vi "LSMcontroller_v61_updatedROIselection.vi"() -> ()   [LabVIEW 2015] (continued)
                    n3057 = Build Path(base path=w6251, name or relative path="subVIs\\Image\\SetROI_v4.vi") -> (appended path=w6249:path)
                    n3058 = call <vilib>:"Set Busy.vi"() -> ("error out"=w6247:errorcluster)  [unwired: 10 in, 1 out]
                    n3059 = Open VI Reference(type specifier VI Refnum (for type only)=refnum<vi> refnum, vi path=w6249, error in (no error)=w6247) -> (vi reference=w6245:refnum<vi>, error out=w6243:errorcluster)  [unwired: 3 in]
                    n3060 = call-by-ref "?"(reference=w6245, error in=w6243) -> (reference out=w6244:refnum<vi>, error out=w6242:errorcluster)  [unwired: 1 in]
                    n3061 = Close Reference(reference=w6244, error in (no error)=w6242) -> (error out=w6246:errorcluster)
                    n3062 = call <vilib>:"Unset Busy.vi"("error in (no error)"=w6246) -> ()  [unwired: 10 in, 1 out]
                    n3063 = local write "status"(w6246) -> ()
                  }
                  frame #2 {
                    n3064 = call "2pparameters.vi"("command"="get") -> ("params out"=w6276:T11)  [unwired: 1 in]
                    n3065 = Unbundle By Name(w6276) -> ("Xpixels Img"=w6275:i32, "Vx-min Img"=w6274:dbl, "VX-max Img"=w6273:dbl, "Ypixels Img"=w6272:i32, "Vy-min Img"=w6271:dbl, "Vy-max Img"=w6270:dbl, "Colormap"=w6269:u16, "square pixels"=w6268:bool, "square matrix"=w6267:bool, "Angle Img"=w6266:dbl, "Drawing Mode"=w6265:u16)
                    n3066 = local write "xpixels ref"(w6275) -> ()
                    n3067 = local write "Vx-min ref"(w6274) -> ()
                    n3068 = local write "Vx-max ref"(w6273) -> ()
                    n3069 = local write "ypixels ref"(w6272) -> ()
                    n3070 = local write "Vy-min ref"(w6271) -> ()
                    n3071 = local write "Vy-max ref"(w6270) -> ()
                    n3072 = local write "Colormap"(w6269) -> ()
                    n3073 = local write "Square pixels"(w6268) -> ()
                    n3074 = local write "square matrix"(w6267) -> ()
                    n3075 = local write "Angle ref"(w6266) -> ()
                    n3076 = local write "ROI Type"(w6265) -> ()
                    n3077 = call "2pparameters.vi"("command"="get") -> ("params out"=w6259:T11)  [unwired: 1 in]
                    n3078 = Unbundle By Name(w6259) -> ("Xpixels"=w6253:i32, "Vxminref"=w6257:dbl, "Vxmaxref"=w6256:dbl, "Ypixels"=w6252:i32, "Vyminref"=w6255:dbl, "Vymaxref"=w6254:dbl, "Colormap"=w6260:u16, "square pixels"=w6261:bool, "square matrix"=w6262:bool, "Angle draw"=w6263:dbl, "Drawing Mode"=w6264:u16)
                    n3079 = local write "Vy-max draw"(w6254) -> ()
                    n3080 = local write "Angle drawing"(w6263) -> ()
                    n3081 = local write "Colormap"(w6260) -> ()
                    n3082 = local write "Square pixels"(w6261) -> ()
                    n3083 = local write "square matrix"(w6262) -> ()
                    n3084 = local write "ROI Type"(w6264) -> ()
                    n3085 = local write "xpixels draw"(w6253) -> ()
                    n3086 = local write "ypixels draw"(w6252) -> ()
                    n3087 = local write "Vx-min draw"(w6257) -> ()
                    n3088 = local write "Vx-max draw"(w6256) -> ()
                    n3089 = local write "Vy-min draw"(w6255) -> ()
                  }
                  frame #3 {
                    n3090 = property on="ROI" class="Bool (strict)"("Val(Sgnl)"=FALSE ("x/y scan")) -> ()  [unwired: 2 in, 2 out]
                  }
                }
              }
            }
          }
          event "Xdattype": Value Change {
            n3091 = event-data() -> ()  [unwired: 1 in, 1 out]
            n3092 = case shown="True" "Xdattype" {
              frame False {
              }
              frame True {
                n3093 = stacked-sequence {
                  frame #0 {
                    n3094 = Current VI's Path() -> (path=w6289:path)
                    n3095 = Strip Path(path=w6289) -> (stripped path=w6290:path)  [unwired: 1 out]
                    n3096 = Build Path(base path=w6290, name or relative path="subVIs\\Misc\\Changedataconfig.vi") -> (appended path=w6288:path)
                    n3097 = call <vilib>:"Set Busy.vi"() -> ("error out"=w6286:errorcluster)  [unwired: 10 in, 1 out]
                    n3098 = Open VI Reference(type specifier VI Refnum (for type only)=refnum<vi> refnum, vi path=w6288, error in (no error)=w6286) -> (vi reference=w6281:refnum<vi>, error out=w6283:errorcluster)  [unwired: 3 in]
                    n3099 = call-by-ref "?"(reference=w6281, error in=w6283) -> (reference out=w6285:refnum<vi>, error out=w6284:errorcluster)  [unwired: 12 in]
                    n3100 = Close Reference(reference=w6285, error in (no error)=w6284) -> (error out=w6280:errorcluster)
                    "status" <- w6280
                    n3101 = call <vilib>:"Unset Busy.vi"("error in (no error)"=w6280) -> ()  [unwired: 10 in, 1 out]
                  }
                  frame #1 {
                    n3102 = property on="Xdattype" class="Bool (strict)"("Val(Sgnl)"=FALSE ("x/y scan")) -> ()  [unwired: 2 in, 2 out]
                  }
                }
              }
            }
          }
          event "XautoOD": Value Change {
            n3103 = event-data() -> ()  [unwired: 1 in, 1 out]
            n3104 = case shown="True" "XautoOD" {
              frame False {
              }
              frame True {
                n3105 = stacked-sequence {
                  frame #0 {
                    n3106 = Current VI's Path() -> (path=w6302:path)
                    n3107 = Strip Path(path=w6302) -> (stripped path=w6303:path)  [unwired: 1 out]
                    n3108 = Build Path(base path=w6303, name or relative path="subVIs\\Misc\\ChangeautoODs.vi") -> (appended path=w6301:path)
                    n3109 = call <vilib>:"Set Busy.vi"() -> ("error out"=w6299:errorcluster)  [unwired: 10 in, 1 out]
                    n3110 = Open VI Reference(type specifier VI Refnum (for type only)=refnum<vi> refnum, vi path=w6301, error in (no error)=w6299) -> (vi reference=w6294:refnum<vi>, error out=w6296:errorcluster)  [unwired: 3 in]
                    n3111 = call-by-ref "?"(reference=w6294, error in=w6296) -> (reference out=w6298:refnum<vi>, error out=w6297:errorcluster)  [unwired: 12 in]
                    n3112 = Close Reference(reference=w6298, error in (no error)=w6297) -> (error out=w6293:errorcluster)
                    "status 2" <- w6293
                    n3113 = call <vilib>:"Unset Busy.vi"("error in (no error)"=w6293) -> ()  [unwired: 10 in, 1 out]
                  }
                  frame #1 {
                    n3114 = property on="XautoOD" class="Bool (strict)"("Val(Sgnl)"=FALSE ("x/y scan")) -> ()  [unwired: 2 in, 2 out]
                  }
                }
              }
            }
          }
          event "SetMan": Value Change {
            n3115 = event-data() -> ()  [unwired: 1 in, 1 out]
            n3116 = case shown="True" "SetMan" {
              frame False {
              }
              frame True {
                n3117 = stacked-sequence {
                  frame #0 {
                    w6306 = u16 0 items=["Rectangle", "Circle", "Freeform Boundary", "Freeform Interior"] ("ROI Type")
                    n3118 = local write "ROI Type"(w6306) -> ()
                    n3119 = local read "Square pixels"() -> (w6312:bool)
                    n3120 = case shown="True" w6312 {
                      frame False {
                        n3121 = local read "square matrix"() -> (w6313:bool)
                        n3122 = case shown="False" w6313 {
                          frame False {
                            "ypixels ref" <- "ypixels"
                            "xpixels ref" <- "xpixels"
                          }
                          frame True {
                            n3123 = local read "xpixels"() -> (w6318:i32)
                            n3124 = local read "ypixels"() -> (w6317:i32)
                            n3125 = Max & Min(x=w6318, y=w6317) -> (max(x,y)=w6316:i32)  [unwired: 1 out]
                            n3126 = local write "xpixels ref"(w6316) -> ()
                            n3127 = local write "ypixels ref"(w6316) -> ()
                          }
                        }
                      }
                      frame True {
                        n3128 = local read "square matrix"() -> (w6319:bool)
                        n3129 = case shown="False" w6319 {
                          frame False {
                            n3130 = local read "Vxmax"() -> (w6333:dbl)
                            n3131 = local read "Vx-min"() -> (w6332:dbl)
                            n3132 = local read "Vy-max"() -> (w6328:dbl)
                            n3133 = local read "Vy-min"() -> (w6329:dbl)
                            n3134 = Subtract(x=w6328, y=w6329) -> (x-y=w6330:dbl)
                            n3135 = Subtract(x=w6333, y=w6332) -> (x-y=w6331:dbl)
                            n3136 = Absolute Value(x=w6330) -> (abs(x)=w6321:dbl)
                            n3137 = Absolute Value(x=w6331) -> (abs(x)=w6322:dbl)
                            n3138 = Divide(x=w6322, y=w6321) -> (x/y=w6327:dbl)
                            n3139 = Greater Or Equal?(x=w6322, y=w6321) -> (x >= y?=w6320:bool)
                            n3140 = local read "xpixels"() -> (w6326:i32)
                            n3141 = local read "ypixels"() -> (w6323:i32)
                            n3142 = case shown="False" w6320 {
                              tunnel: w6327 -> [w6338 w6341]
                              tunnel: w6326 -> [w6335 _]
                              tunnel: [w6335 w6340] -> w6325
                              tunnel: [w6334 w6339] -> w6324
                              tunnel: w6323 -> [_ w6339]
                              frame False {
                                n3143 = To Double Precision Float(number=w6335) -> (double precision float=w6337:dbl)
                                n3144 = Divide(x=w6337, y=w6338) -> (x/y=w6336:dbl)
                                n3145 = To Long Integer(number=w6336) -> (32bit integer=w6334:i32)
                              }
                              frame True {
                                n3146 = To Double Precision Float(number=w6339) -> (double precision float=w6343:dbl)
                                n3147 = Multiply(x=w6343, y=w6341) -> (x*y=w6342:dbl)
                                n3148 = To Long Integer(number=w6342) -> (32bit integer=w6340:i32)
                              }
                            }
                            n3149 = local write "ypixels ref"(w6324) -> ()
                            n3150 = local write "xpixels ref"(w6325) -> ()
                          }
                          frame True {
                          }
                        }
                      }
                    }
                    "Vx-max ref" <- "Vxmax"
                    "Vx-min ref" <- "Vx-min"
                    "Vy-max ref" <- "Vy-max"
                    "Vy-min ref" <- "Vy-min"
                    "Angle ref" <- "Angle"
                  }
                  frame #1 {
                    n3151 = property on="SetMan" class="Bool (strict)"("Val(Sgnl)"=FALSE ("Value (Signaling)")) -> ()  [unwired: 2 in, 2 out]
                  }
                }
              }
            }
          }
          event "SetMan 2": Value Change {
            n3152 = event-data() -> ()  [unwired: 1 in, 1 out]
            n3153 = case shown="True" "SetMan 2" {
              frame False {
              }
              frame True {
                n3154 = stacked-sequence {
                  frame #0 {
                    n3155 = local write "Vx-ref"("Vx") -> ()
                    n3156 = local write "Vy-ref"("Vy") -> ()
                  }
                  frame #1 {
                    n3157 = property on="SetMan 2" class="Bool (strict)"("Val(Sgnl)"=FALSE ("Value (Signaling)")) -> ()  [unwired: 2 in, 2 out]
                  }
                }
              }
            }
          }
          event "Reset Coords": Value Change {
            n3158 = event-data() -> ("NewVal"=w6349:bool)  [unwired: 1 in, 5 out]
            n3159 = case shown="True" w6349 {
              frame False {
              }
              frame True {
                n3160 = stacked-sequence {
                  frame #0 {
                    n3161 = local write "xpixels"(256 ("xpixels")) -> ()
                    n3162 = local write "ypixels"(256 ("ypixels")) -> ()
                    n3163 = local write "Vxmax"(9.0 ("Vx-max")) -> ()
                    n3164 = local write "Vx-min"(-9.0 ("Vx-min")) -> ()
                    n3165 = local write "Vy-max"(9.0 ("Vy-max")) -> ()
                    n3166 = local write "Vy-min"(-9.0 ("Vy-min")) -> ()
                    n3167 = local write "Angle"(0.0 ("Angle")) -> ()
                  }
                  frame #1 {
                    n3168 = property on="Reset Coords" class="Bool (strict)"("Value"=FALSE ("TROI")) -> ()  [unwired: 2 in, 2 out]
                  }
                }
              }
            }
          }
          event "TROI": Value Change {
            n3169 = event-data() -> ()  [unwired: 1 in, 1 out]
            n3170 = case shown="True" "TROI" {
              frame False {
              }
              frame True {
                n3171 = stacked-sequence {
                  frame #0 {
                    n3172 = local read "Vy-min ref"() -> (w6363:dbl)
                    n3173 = local read "Vy-max ref"() -> (w6362:dbl)
                    n3174 = local read "Vx-max ref"() -> (w6360:dbl)
                    n3175 = local read "Vx-min ref"() -> (w6361:dbl)
                    n3176 = local read "ypixels ref"() -> (w6365:i32)
                    n3177 = local read "xpixels ref"() -> (w6364:i32)
                    n3178 = local read "Angle ref"() -> (w6359:dbl)
                    n3179 = local write "Angle"(w6359) -> ()
                    n3180 = local write "xpixels"(w6364) -> ()
                    n3181 = local write "Vy-min"(w6363) -> ()
                    n3182 = local write "Vy-max"(w6362) -> ()
                    n3183 = local write "Vx-min"(w6361) -> ()
                    n3184 = local write "ypixels"(w6365) -> ()
                    n3185 = local write "Vxmax"(w6360) -> ()
                  }
                  frame #1 {
                    n3186 = property on="TROI" class="Bool (strict)"("Value"=FALSE ("TROI")) -> ()  [unwired: 2 in, 2 out]
                  }
                }
              }
            }
          }
          event "TROI 2": Value Change {
            n3187 = event-data() -> ()  [unwired: 1 in, 1 out]
            n3188 = case shown="True" "TROI 2" {
              frame False {
              }
              frame True {
                n3189 = stacked-sequence {
                  frame #0 {
                    n3190 = local read "Vx-ref"() -> (w6368:dbl)
                    n3191 = local read "Vy-ref"() -> (w6369:dbl)
                    n3192 = local write "Vx"(w6368) -> ()
                    n3193 = local write "Vy"(w6369) -> ()
                  }
                  frame #1 {
                    n3194 = property on="TROI 2" class="Bool (strict)"("Value"=FALSE ("TROI")) -> ()  [unwired: 2 in, 2 out]
                  }
                }
              }
            }
          }
          event "Square pixels": Value Change {
            n3195 = event-data() -> ()  [unwired: 1 in, 1 out]
            n3196 = case shown="True" "Square pixels" {
              frame False {
              }
              frame True {
                n3197 = property on="square matrix" class="Bool (strict)"("Value"=FALSE ("square matrix")) -> ()  [unwired: 2 in, 2 out]
                n3198 = property on="Square pixels" class="Bool (strict)"("Value"=TRUE ("square matrix")) -> ()  [unwired: 2 in, 2 out]
              }
            }
          }
          event "square matrix": Value Change {
            n3199 = event-data() -> ()  [unwired: 1 in, 1 out]
            n3200 = case shown="True" "square matrix" {
              frame False {
              }
              frame True {
                n3201 = property on="square matrix" class="Bool (strict)"("Value"=TRUE ("square matrix")) -> ()  [unwired: 2 in, 2 out]
                n3202 = property on="Square pixels" class="Bool (strict)"("Value"=FALSE ("square matrix")) -> ()  [unwired: 2 in, 2 out]
              }
            }
          }
          event "up", "downright", "down", "downleft", "right", "left", "upright", "upleft": Value Change {
            n3203 = event-data() -> ()  [unwired: 1 in, 6 out]
            n3204 = local read "downright"() -> (w6382:bool)
            n3205 = local read "downleft"() -> (w6384:bool)
            n3206 = local read "upright"() -> (w6380:bool)
            n3207 = local read "upleft"() -> (w6378:bool)
            n3208 = local read "down"() -> (w6383:bool)
            n3209 = local read "right"() -> (w6381:bool)
            n3210 = local read "left"() -> (w6385:bool)
            n3211 = local read "up"() -> (w6379:bool)
            n3212 = Compound Arithmetic op=OR(w6378, w6379, w6380, w6381, w6382, w6383, w6384, w6385) -> (w6377:bool)
            n3213 = case shown="True" w6377 {
              frame False {
              }
              frame True {
                n3214 = stacked-sequence {
                  frame #0 {
                    n3215 = local read "downright"() -> (w6387:bool)
                    n3216 = local read "downleft"() -> (w6389:bool)
                    n3217 = local read "BigSmall"() -> (w6386:bool)
                    n3218 = local read "upright"() -> (w6391:bool)
                    n3219 = local read "upleft"() -> (w6394:bool)
                    n3220 = local read "down"() -> (w6390:bool)
                    n3221 = local read "right"() -> (w6392:bool)
                    n3222 = local read "left"() -> (w6388:bool)
                    n3223 = local read "up"() -> (w6393:bool)
                    n3224 = call "movestageparams.vi"("command"="get") -> ("Params out"=w6397:T21)  [unwired: 1 in]
                    n3225 = Bundle By Name(cluster=w6397, "upleft"=w6394, "up"=w6393, "upright"=w6391, "right"=w6392, "downright"=w6387, "down"=w6390, "downleft"=w6389, "left"=w6388, "Bigsmall"=w6386) -> (w6398:T21)
                    n3226 = call "movestageparams.vi"("Params in"=w6398, "command"="set") -> ()  [unwired: 1 out]
                  }
                  frame #1 {
                    n3227 = disable-structure shown="Disabled" {
                      frame Disabled {
                        n3228 = call "configuration.vi"("command"="get") -> ("config out"=w6401:T12)  [unwired: 2 in, 1 out]
                        n3229 = in-place {
                          n3230 = in-place-cluster #45(w6401) -> ()  [unwired: 2 out]
                          n3231 = in-place-cluster #45("StageL"="StageL", "StageS"="StageS") -> (w6399:T12)
                        }
                        n3232 = call "configuration.vi"("config in"=w6399, "command"="set") -> ()  [unwired: 1 in, 2 out]
                      }
                      frame Enabled {
                      }
                    }
                  }
                  frame #2 {
                    n3233 = call "movestage.vi"() -> ()  [unwired: 12 in]
                  }
                  frame #3 {
                    w6405 = FALSE ("OK Button")
                    w6406 = FALSE ("OK Button")
                    n3234 = property on="down" class="Bool (strict)"("Value"=w6406) -> ()  [unwired: 2 in, 2 out]
                    n3235 = property on="up" class="Bool (strict)"("Value"=w6406) -> ()  [unwired: 2 in, 2 out]
                    n3236 = property on="right" class="Bool (strict)"("Value"=w6406) -> ()  [unwired: 2 in, 2 out]
                    n3237 = property on="left" class="Bool (strict)"("Value"=w6406) -> ()  [unwired: 2 in, 2 out]
                    n3238 = property on="upright" class="Bool (strict)"("Value"=w6405) -> ()  [unwired: 2 in, 2 out]
                    n3239 = property on="downleft" class="Bool (strict)"("Value"=w6405) -> ()  [unwired: 2 in, 2 out]
                    n3240 = property on="downright" class="Bool (strict)"("Value"=w6405) -> ()  [unwired: 2 in, 2 out]
                    n3241 = property on="upleft" class="Bool (strict)"("Value"=w6405) -> ()  [unwired: 2 in, 2 out]
                  }
                }
              }
            }
          }
          event "finite samples": Value Change {
            n3242 = event-data() -> ("NewVal"=w6407:bool)  [unwired: 1 in]
            n3243 = flat-sequence {
              tunnel: w6407 -> [w6408]
              frame #0 {
                n3244 = case shown="True" w6408 {
                  frame False {
                    w6409 = FALSE ("wavdet")
                    n3245 = property on="continuous" class="Bool (strict)"("Value"=TRUE ("continuous for display")) -> ()  [unwired: 2 in, 2 out]
                    n3246 = property on="wavdet" class="Bool (strict)"("Value"=w6409) -> ()  [unwired: 2 in, 2 out]
                    n3247 = property on="save\ndata" class="Bool (strict)"("Value"=w6409) -> ()  [unwired: 2 in, 2 out]
                    n3248 = property on="# of frames" class="DigNum (strict)"("DisabledEnum"=T7."Disabled and Grayed Out" ("Disabled")) -> ()  [unwired: 2 in, 2 out]
                    n3249 = property on="save\ndata" class="Bool (strict)"("DisabledEnum"=T7."Disabled and Grayed Out" ("Disabled")) -> ()  [unwired: 2 in, 2 out]
                    "Save tab" <- enum32{"withsave", "withoutsave"}."withsave" ("Save tab")
                  }
                  frame True {
                    w6416 = FALSE ("continuous for display")
                    n3250 = property on="continuous" class="Bool (strict)"("Value"=w6416) -> ()  [unwired: 2 in, 2 out]
                    n3251 = property on="wavdet" class="Bool (strict)"("Value"=w6416) -> ()  [unwired: 2 in, 2 out]
                    n3252 = local write "Save tab"(enum32{"withsave", "withoutsave"}."withsave" ("Save tab")) -> ()
                    n3253 = property on="save\ndata" class="Bool (strict)"("DisabledEnum"=T7."Enabled" ("Disabled")) -> ()  [unwired: 2 in, 2 out]
                    n3254 = property on="save\ndata" class="Bool (strict)"("Value"=TRUE ("save\ndata")) -> ()  [unwired: 2 in, 2 out]
                    n3255 = property on="# of frames" class="DigNum (strict)"("DisabledEnum"=T7."Enabled" ("Disabled")) -> ()  [unwired: 2 in, 2 out]
                  }
                }
              }
              frame #1 {
                n3256 = local read "finite samples"() -> (w6425:bool)
                n3257 = local read "continuous"() -> (w6424:bool)
                n3258 = local read "wavdet"() -> (w6423:bool)
                n3259 = call "2pparameters.vi"("command"="get") -> ("params out"=w6419:T11)  [unwired: 1 in]
                n3260 = Bundle By Name(cluster=w6419, "finite"=w6425, "cont"=w6424, "wavdet"=w6423) -> (w6422:T11)
                n3261 = call "2pparameters.vi"("Params in"=w6422, "command"="set") -> ()  [unwired: 1 out]
              }
            }
          }
          event "continuous": Value Change {
            n3262 = event-data() -> ("NewVal"=w6426:bool)  [unwired: 1 in]
            n3263 = flat-sequence {
              tunnel: w6426 -> [w6427]
              frame #0 {
                n3264 = case shown="True" w6427 {
                  frame False {
                    n3265 = property on="finite samples" class="Bool (strict)"("Value"=TRUE ("finite samples for recording")) -> ()  [unwired: 2 in, 2 out]
                    n3266 = property on="save\ndata" class="Bool (strict)"("Value"=TRUE ("save\ndata")) -> ()  [unwired: 2 in, 2 out]
                    n3267 = property on="wavdet" class="Bool (strict)"("Value"=FALSE ("wavdet")) -> ()  [unwired: 2 in, 2 out]
                    n3268 = local write "Save tab"(enum32{"withsave", "withoutsave"}."withsave" ("Save tab")) -> ()
                    n3269 = property on="# of frames" class="DigNum (strict)"("DisabledEnum"=T7."Enabled" ("Disabled")) -> ()  [unwired: 2 in, 2 out]
                    n3270 = property on="save\ndata" class="Bool (strict)"("DisabledEnum"=T7."Enabled" ("Disabled")) -> ()  [unwired: 2 in, 2 out]
                  }
                  frame True {
                    w6434 = FALSE ("finite samples for recording")
                    n3271 = property on="finite samples" class="Bool (strict)"("Value"=w6434) -> ()  [unwired: 2 in, 2 out]
                    n3272 = property on="wavdet" class="Bool (strict)"("Value"=w6434) -> ()  [unwired: 2 in, 2 out]
                    n3273 = property on="save\ndata" class="Bool (strict)"("Value"=w6434) -> ()  [unwired: 2 in, 2 out]
                    n3274 = local write "Save tab"(enum32{"withsave", "withoutsave"}."withsave" ("Save tab")) -> ()
                    n3275 = property on="# of frames" class="DigNum (strict)"("DisabledEnum"=T7."Disabled and Grayed Out" ("Disabled")) -> ()  [unwired: 2 in, 2 out]
                    n3276 = property on="save\ndata" class="Bool (strict)"("DisabledEnum"=T7."Disabled and Grayed Out" ("Disabled")) -> ()  [unwired: 2 in, 2 out]
                  }
                }
              }
              frame #1 {
                n3277 = local read "finite samples"() -> (w6444:bool)
                n3278 = local read "continuous"() -> (w6443:bool)
                n3279 = local read "wavdet"() -> (w6442:bool)
                n3280 = call "2pparameters.vi"("command"="get") -> ("params out"=w6438:T11)  [unwired: 1 in]
                n3281 = Bundle By Name(cluster=w6438, "finite"=w6444, "cont"=w6443, "wavdet"=w6442) -> (w6441:T11)
                n3282 = call "2pparameters.vi"("Params in"=w6441, "command"="set") -> ()  [unwired: 1 out]
              }
            }
          }
          event "wavdet": Value Change {
            n3283 = event-data() -> ("NewVal"=w6445:bool)  [unwired: 1 in]
            n3284 = flat-sequence {
              tunnel: w6445 -> [w6446]
              frame #0 {
                n3285 = case shown="False" w6446 {
                  frame False {
                    n3286 = property on="finite samples" class="Bool (strict)"("Value"=TRUE ("finite samples for recording")) -> ()  [unwired: 2 in, 2 out]
                    n3287 = property on="continuous" class="Bool (strict)"("Value"=FALSE ("continuous")) -> ()  [unwired: 2 in, 2 out]
                    n3288 = local write "Save tab"(enum32{"withsave", "withoutsave"}."withsave" ("Save tab")) -> ()
                    n3289 = property on="save\ndata" class="Bool (strict)"("DisabledEnum"=T7."Enabled" ("Disabled")) -> ()  [unwired: 2 in, 2 out]
                    n3290 = property on="# of frames" class="DigNum (strict)"("DisabledEnum"=T7."Enabled" ("Disabled")) -> ()  [unwired: 2 in, 2 out]
                    n3291 = property on="save\ndata" class="Bool (strict)"("Value"=TRUE ("save\ndata")) -> ()  [unwired: 2 in, 2 out]
                  }
                  frame True {
                    w6455 = FALSE ("finite samples for recording")
                    n3292 = property on="finite samples" class="Bool (strict)"("Value"=w6455) -> ()  [unwired: 2 in, 2 out]
                    n3293 = property on="continuous" class="Bool (strict)"("Value"=w6455) -> ()  [unwired: 2 in, 2 out]
                    n3294 = property on="save\ndata" class="Bool (strict)"("DisabledEnum"=T7."Enabled" ("Disabled")) -> ()  [unwired: 2 in, 2 out]
                    n3295 = local write "Save tab"(enum32{"withsave", "withoutsave"}."withsave" ("Save tab")) -> ()
                    n3296 = property on="# of frames" class="DigNum (strict)"("DisabledEnum"=T7."Disabled" ("Disabled")) -> ()  [unwired: 2 in, 2 out]
                    n3297 = property on="save\ndata" class="Bool (strict)"("Value"=TRUE ("save\ndata")) -> ()  [unwired: 2 in, 2 out]
                  }
                }
              }
              frame #1 {
                n3298 = local read "finite samples"() -> (w6458:bool)
                n3299 = local read "continuous"() -> (w6459:bool)
                n3300 = local read "wavdet"() -> (w6460:bool)
                n3301 = call "2pparameters.vi"("command"="get") -> ("params out"=w6464:T11)  [unwired: 1 in]
                n3302 = Bundle By Name(cluster=w6464, "finite"=w6458, "cont"=w6459, "wavdet"=w6460) -> (w6461:T11)
                n3303 = call "2pparameters.vi"("Params in"=w6461, "command"="set") -> ()  [unwired: 1 out]
              }
            }
          }
          event "cursors": Value Change {
            n3304 = event-data() -> ()  [unwired: 1 in, 5 out]
            n3305 = case shown="True" "cursors" {
              frame False {
                n3306 = property on="img_CH1" class="IntGraph (strict)"("Active Cursor"=u32 0, "Cursor.Cursor Style"=u8 0 ("Cursor Style"), "Cursor.Cursor Point Style"=u8 0 ("Cursor Point Style")) -> ("Cursor.Cursor Position:Cursor X"=w6469:dbl, "Cursor.Cursor Position:Cursor Y"=w6470:dbl)  [unwired: 2 in, 2 out]
                n3307 = property on="img_CH2" class="IntGraph (strict)"("Active Cursor"=u32 0, "Cursor.Cursor Style"=u8 0 ("Cursor Style"), "Cursor.Cursor Point Style"=u8 0 ("Cursor Point Style")) -> ()  [unwired: 2 in, 2 out]
                n3308 = local write "cursor x [pixel]"(w6469) -> ()
                n3309 = local write "cursor y [pixel]"(w6470) -> ()
              }
              frame True {
                n3310 = stacked-sequence {
                  frame #0 {
                    n3311 = call "2pparameters.vi"("command"="get") -> ("params out"=w6485:T11)  [unwired: 1 in]
                    n3312 = Unbundle By Name(w6485) -> ("Xpixels Img"=w6486:i32, "Ypixels Img"=w6483:i32)
                    n3313 = To Double Precision Float(number=w6483) -> (double precision float=w6477:dbl)
                    n3314 = To Double Precision Float(number=w6486) -> (double precision float=w6482:dbl)
                    n3315 = Divide(x=w6477, y=2.0) -> (x/y=w6478:dbl)
                    n3316 = Divide(x=w6482, y=2.0) -> (x/y=w6480:dbl)
                    n3317 = Round To Nearest(number=w6478) -> (nearest integer value=w6476:dbl)
                    n3318 = Round To Nearest(number=w6480) -> (nearest integer value=w6479:dbl)
                    n3319 = property on="img_CH1" class="IntGraph (strict)"("Active Cursor"=u32 0, "Cursor.Cursor Style"=u8 8 ("Cursor Style"), "Cursor.Cursor Point Style"=u8 5 ("Cursor Point Style"), "Cursor.Cursor Position:Cursor X"=w6479, "Cursor.Cursor Position:Cursor Y"=w6476, "Cursor.Visible"=TRUE) -> ()  [unwired: 2 in, 2 out]
                  }
                  frame #1 {
                    n3320 = call "2pparameters.vi"("command"="get") -> ("params out"=w6505:T11)  [unwired: 1 in]
                    n3321 = call "2pparameters.vi"("command"="get") -> ("params out"=w6503:T11)  [unwired: 1 in]
                    n3322 = property on="img_CH1" class="IntGraph (strict)"("Active Cursor"=u32 0, "Cursor.Cursor Style"=u8 8 ("Cursor Style"), "Cursor.Cursor Point Style"=u8 5 ("Cursor Point Style")) -> ("Cursor.Cursor Position:Cursor X"=w6498:dbl, "Cursor.Cursor Position:Cursor Y"=w6497:dbl, "Cursor.Cursor Index"=w6520:i32, "Cursor.Cursor Plot"=w6519:i32, "Cursor.Visible"=w6490:bool)  [unwired: 2 in, 2 out]
                    "cursor x [pixel]" <- w6498
                    "cursor y [pixel]" <- w6497
                    n3323 = Unbundle By Name(w6505) -> ("Vy-max Img"=w6507:dbl, "Vy-min Img"=w6494:dbl, "Ypixels Img"=w6509:i32)
                    n3324 = Unbundle By Name(w6503) -> ("VX-max Img"=w6504:dbl, "Vx-min Img"=w6492:dbl, "Xpixels Img"=w6508:i32)
                    n3325 = Subtract(x=w6507, y=w6494) -> (x-y=w6512:dbl)
                    n3326 = Subtract(x=w6504, y=w6492) -> (x-y=w6510:dbl)
                    n3327 = local read "img_CH2"() -> (w6516:sgl[][])
                    n3328 = To Double Precision Float(number=w6508) -> (double precision float=w6511:dbl)
                    n3329 = local read "img_CH1"() -> (w6517:sgl[][])
                    n3330 = To Double Precision Float(number=w6509) -> (double precision float=w6513:dbl)
                    n3331 = Index Array(array=w6517, index (row)=w6520, index (col)=w6519) -> (element=→"value CH 1":sgl)
                    n3332 = Index Array(array=w6516, index (row)=w6520, index (col)=w6519) -> (element=→"value CH 2":sgl)
                    n3333 = Divide(x=w6510, y=w6511) -> (x/y=w6514:dbl)
                    n3334 = Divide(x=w6512, y=w6513) -> (x/y=w6515:dbl)
                    n3335 = Multiply(x=w6498, y=w6514) -> (x*y=w6493:dbl)
                    n3336 = Multiply(x=w6497, y=w6515) -> (x*y=w6496:dbl)
                    n3337 = property on="img_CH2" class="IntGraph (strict)"("Active Cursor"=u32 0, "Cursor.Cursor Style"=u8 8 ("Cursor Style"), "Cursor.Cursor Point Style"=u8 5 ("Cursor Point Style"), "Cursor.Cursor Position:Cursor X"=w6498, "Cursor.Cursor Position:Cursor Y"=w6497, "Cursor.Visible"=w6490) -> ()  [unwired: 2 in, 2 out]
                    n3338 = Add(x=w6493, y=w6492) -> (x+y=w6491:dbl)
                    n3339 = Add(x=w6496, y=w6494) -> (x+y=w6495:dbl)
                    n3340 = local write "Vx-ref"(w6491) -> ()
                    n3341 = local write "Vy-ref"(w6495) -> ()
                  }
                }
              }
            }
          }
          event "img_CH1": Cursor Move {
            n3342 = event-data() -> ("CursIdx"=w6525:i32)  [unwired: 1 in]
            n3343 = Equal To 0?(x=w6525) -> (x = 0?=w6526:bool)
            n3344 = case shown="True" w6526 {
              frame False {
              }
              frame True {
                n3345 = call "2pparameters.vi"("command"="get") -> ("params out"=w6546:T11)  [unwired: 1 in]
                n3346 = call "2pparameters.vi"("command"="get") -> ("params out"=w6548:T11)  [unwired: 1 in]
                n3347 = property on="img_CH1" class="IntGraph (strict)"("Active Cursor"=u32 0, "Cursor.Cursor Style"=u8 8 ("Cursor Style"), "Cursor.Cursor Point Style"=u8 5 ("Cursor Point Style")) -> ("Cursor.Cursor Position:Cursor X"=w6535:dbl, "Cursor.Cursor Position:Cursor Y"=w6534:dbl, "Cursor.Cursor Plot"=w6554:i32, "Cursor.Cursor Index"=w6553:i32, "Cursor.Visible"=w6527:bool)  [unwired: 2 in, 2 out]
                n3348 = Unbundle By Name(w6546) -> ("Vy-max Img"=w6544:dbl, "Vy-min Img"=w6533:dbl, "Ypixels Img"=w6542:i32)
                n3349 = Unbundle By Name(w6548) -> ("VX-max Img"=w6547:dbl, "Vx-min Img"=w6528:dbl, "Xpixels Img"=w6543:i32)
                n3350 = Subtract(x=w6544, y=w6533) -> (x-y=w6539:dbl)
                n3351 = Subtract(x=w6547, y=w6528) -> (x-y=w6541:dbl)
                n3352 = local write "cursor x [pixel]"(w6535) -> ()
                n3353 = local write "cursor y [pixel]"(w6534) -> ()
                n3354 = To Double Precision Float(number=w6543) -> (double precision float=w6540:dbl)
                n3355 = To Double Precision Float(number=w6542) -> (double precision float=w6538:dbl)
                n3356 = local read "img_CH2"() -> (w6555:sgl[][])
                n3357 = local read "img_CH1"() -> (w6558:sgl[][])
                n3358 = Index Array(array=w6555, index (row)=w6554, index (col)=w6553) -> (element=w6556:sgl)
                n3359 = Index Array(array=w6558, index (row)=w6554, index (col)=w6553) -> (element=w6557:sgl)
                n3360 = Divide(x=w6541, y=w6540) -> (x/y=w6537:dbl)
                n3361 = Divide(x=w6539, y=w6538) -> (x/y=w6536:dbl)
                n3362 = local write "value CH 2"(w6556) -> ()
                n3363 = Multiply(x=w6535, y=w6537) -> (x*y=w6530:dbl)
                n3364 = local write "value CH 1"(w6557) -> ()
                n3365 = Multiply(x=w6534, y=w6536) -> (x*y=w6532:dbl)
                n3366 = Add(x=w6530, y=w6528) -> (x+y=w6529:dbl)
                n3367 = local write "Vx-ref"(w6529) -> ()
                n3368 = Add(x=w6532, y=w6533) -> (x+y=w6531:dbl)
                n3369 = property on="img_CH2" class="IntGraph (strict)"("Active Cursor"=u32 0, "Cursor.Cursor Style"=u8 8 ("Cursor Style"), "Cursor.Cursor Point Style"=u8 5 ("Cursor Point Style"), "Cursor.Cursor Position:Cursor X"=w6535, "Cursor.Cursor Position:Cursor Y"=w6534, "Cursor.Visible"=w6527) -> ()  [unwired: 2 in, 2 out]
                n3370 = local write "Vy-ref"(w6531) -> ()
              }
            }
          }
          event "img_CH2": Cursor Move {
            n3371 = event-data() -> ("CursIdx"=w6562:i32)  [unwired: 1 in]
            n3372 = Equal To 0?(x=w6562) -> (x = 0?=w6563:bool)
            n3373 = case shown="True" w6563 {
              frame False {
              }
              frame True {
                n3374 = property on="img_CH2" class="IntGraph (strict)"("Active Cursor"=u32 0, "Cursor.Cursor Style"=u8 8 ("Cursor Style"), "Cursor.Cursor Point Style"=u8 5 ("Cursor Point Style")) -> ("Cursor.Cursor Position:Cursor X"=w6571:dbl, "Cursor.Cursor Position:Cursor Y"=w6572:dbl, "Cursor.Cursor Plot"=w6591:i32, "Cursor.Cursor Index"=w6590:i32, "Cursor.Visible"=w6564:bool)  [unwired: 2 in, 2 out]
                n3375 = call "2pparameters.vi"("command"="get") -> ("params out"=w6583:T11)  [unwired: 1 in]
                n3376 = call "2pparameters.vi"("command"="get") -> ("params out"=w6585:T11)  [unwired: 1 in]
                n3377 = local read "img_CH1"() -> (w6595:sgl[][])
                n3378 = local read "img_CH2"() -> (w6592:sgl[][])
                n3379 = local write "cursor x [pixel]"(w6571) -> ()
                n3380 = local write "cursor y [pixel]"(w6572) -> ()
                n3381 = Unbundle By Name(w6583) -> ("Vy-max Img"=w6581:dbl, "Vy-min Img"=w6566:dbl, "Ypixels Img"=w6579:i32)
                n3382 = Unbundle By Name(w6585) -> ("VX-max Img"=w6584:dbl, "Vx-min Img"=w6569:dbl, "Xpixels Img"=w6580:i32)
                n3383 = Index Array(array=w6595, index (row)=w6591, index (col)=w6590) -> (element=w6594:sgl)
                n3384 = Index Array(array=w6592, index (row)=w6591, index (col)=w6590) -> (element=w6593:sgl)
                n3385 = local write "value CH 2"(w6593) -> ()
                n3386 = local write "value CH 1"(w6594) -> ()
                n3387 = Subtract(x=w6581, y=w6566) -> (x-y=w6576:dbl)
                n3388 = Subtract(x=w6584, y=w6569) -> (x-y=w6578:dbl)
                n3389 = To Double Precision Float(number=w6580) -> (double precision float=w6577:dbl)
                n3390 = To Double Precision Float(number=w6579) -> (double precision float=w6575:dbl)
                n3391 = Divide(x=w6578, y=w6577) -> (x/y=w6574:dbl)
                n3392 = Divide(x=w6576, y=w6575) -> (x/y=w6573:dbl)
                n3393 = Multiply(x=w6571, y=w6574) -> (x*y=w6570:dbl)
                n3394 = Multiply(x=w6572, y=w6573) -> (x*y=w6567:dbl)
                n3395 = property on="img_CH1" class="IntGraph (strict)"("Active Cursor"=u32 0, "Cursor.Cursor Style"=u8 8 ("Cursor Style"), "Cursor.Cursor Point Style"=u8 5 ("Cursor Point Style"), "Cursor.Cursor Position:Cursor X"=w6571, "Cursor.Cursor Position:Cursor Y"=w6572, "Cursor.Visible"=w6564) -> ()  [unwired: 2 in, 2 out]
                n3396 = Add(x=w6570, y=w6569) -> (x+y=→"Vx-ref":dbl)
                n3397 = Add(x=w6567, y=w6566) -> (x+y=→"Vy-ref":dbl)
              }
            }
          }
          event "auto shutter": Value Change {
            n3398 = event-data() -> ()  [unwired: 1 in, 6 out]
            n3399 = call "2pparameters.vi"("command"="get") -> ("params out"=w6601:T11)  [unwired: 1 in]
            n3400 = in-place {
              n3401 = in-place-cluster #46(w6601) -> ()  [unwired: 1 out]
              n3402 = local read "auto shutter"() -> (w6603:bool)
              n3403 = in-place-cluster #46("autoshutter"=w6603) -> (w6599:T11)
            }
            n3404 = call "2pparameters.vi"("Params in"=w6599, "command"="set") -> ()  [unwired: 1 out]
          }
          event "auto OD": Value Change {
            n3405 = event-data() -> ()  [unwired: 1 in, 6 out]
            n3406 = call "2pparameters.vi"("command"="get") -> ("params out"=w6606:T11)  [unwired: 1 in]
            n3407 = in-place {
              n3408 = in-place-cluster #47(w6606) -> ()  [unwired: 1 out]
              n3409 = local read "auto OD"() -> (w6608:bool)
              n3410 = in-place-cluster #47("auto OD"=w6608) -> (w6604:T11)
            }
            n3411 = call "2pparameters.vi"("Params in"=w6604, "command"="set") -> ()  [unwired: 1 out]
          }
          event "ODfilt": Value Change {
            n3412 = event-data() -> ("OldVal"=w6609:u16)  [unwired: 1 in, 5 out]
            n3413 = local read "ODfilt"() -> (w6610:u16)
            n3414 = call "2pparameters.vi"("command"="get") -> ("params out"=w6613:T11)  [unwired: 1 in]
            n3415 = call "filterwheelcontrol_nothorlabslib.vi"("Current OD filt"=w6609, "New ODfilt"=w6610) -> ()  [unwired: 1 in]
            n3416 = in-place {
              in-place-border: w6610 -> [w6615]
              n3417 = in-place-cluster #48(w6613) -> ()  [unwired: 1 out]
              n3418 = in-place-cluster #48("ODfilt"=w6615) -> (w6611:T11)
            }
            n3419 = call "2pparameters.vi"("Params in"=w6611, "command"="set") -> ()  [unwired: 1 out]
          }
          event "Exit": Value Change {
            n3420 = event-data() -> ()  [unwired: 1 in, 5 out]
          }
        }
        n3421 = Wait (ms)(milliseconds to wait=u32 50) -> ()  [unwired: 1 out]
      }
      n3422 = while {
        stop <- w69 stop-if-true
        # "Waveform generation"
        n3423 = event shown="[2] \"AO channels\": Value Change" {
          selector: _ -> [_ _ _ _ _ _ _ _ _ _ _ _ _ _ _ _ _]
          dyn-events: _ -> [_ _ _ _ _ _ _ _ _ _ _ _ _ _ _ _ _]
          timeout: _ -> [_ _ _ _ _ _ _ _ _ _ _ _ _ _ _ _ _]
          tunnel: [_ _ _ _ _ _ _ _ _ _ _ _ _ _ _ _ w2042] -> w69
          event Timeout {
            n3424 = event-data() -> ()  [unwired: 1 in, 3 out]
          }
          event "Add AO wave": Value Change {
            n3425 = event-data() -> ("NewVal"=w70:bool)  [unwired: 1 in, 5 out]
            n3426 = case shown="True" w70 {
              frame False {
              }
              frame True {
                n3427 = stacked-sequence {
                  frame #0 {
                    n3428 = local read "Measurement"() -> (w71:T4)
                    n3429 = case shown="\"Lifetime (contour)\"" w71 {
                      frame "X-Y-t movie", Default {
                        n3430 = local read "avpp"() -> (w92:i32)
                        n3431 = local read "Angle ref"() -> (w91:dbl)
                        n3432 = local read "ROI Type"() -> (w90:u16)
                        n3433 = local read "xpixels ref"() -> (w87:i32)
                        n3434 = local read "Vx-min ref"() -> (w86:dbl)
                        n3435 = local read "Vx-max ref"() -> (w85:dbl)
                        n3436 = local read "ypixels ref"() -> (w83:i32)
                        n3437 = local read "Vy-min ref"() -> (w84:dbl)
                        n3438 = local read "Vy-max ref"() -> (w80:dbl)
                        n3439 = local read "Sampling rate"() -> (w74:dbl)
                        n3440 = local read "finite samples"() -> (w75:bool)
                        n3441 = local read "continuous"() -> (w78:bool)
                        n3442 = local read "wavdet"() -> (w79:bool)
                        n3443 = local read "# of frames"() -> (w77:i32)
                        n3444 = local read "maxbufferAI"() -> (w76:i32)
                        n3445 = local read "Override AI buffer"() -> (w72:bool)
                        n3446 = call "2pparameters.vi"("command"="get") -> ("params out"=w89:T11)  [unwired: 1 in]
                        n3447 = Bundle By Name(cluster=w89, "type"="X-Y-t movie", "avpp"=w92, "Angle Img"=w91, "Xpixels Img"=w87, "Vx-min Img"=w86, "VX-max Img"=w85, "Ypixels Img"=w83, "Vy-min Img"=w84, "Vy-max Img"=w80, "srate"=w74, "srate Img"=w74, "finite"=w75, "cont"=w78, "wavdet"=w79, "measpoints"=w77, "maxbufferAI"=w76, "Drawing Mode"=w90, "Vz-reset"=0.0, "AIoverride"=w72) -> (w81:T11)
                        n3448 = call "2pparameters.vi"("Params in"=w81, "command"="set") -> ()  [unwired: 1 out]
                      }
                      frame "X-Y-Z stack" {
                        n3449 = call "2pparameters.vi"("command"="get") -> ("params out"=w96:T11)  [unwired: 1 in]
                        n3450 = Bundle By Name(cluster=w96, "type"="X-Y-Z stack") -> (w94:T11)
                        n3451 = call "2pparameters.vi"("Params in"=w94, "command"="set") -> ()  [unwired: 1 out]
                      }
                      frame "Lifetime (scan)" {
                        n3452 = call "2pparameters.vi"("command"="get") -> ("params out"=w101:T11)  [unwired: 1 in]
                        n3453 = Bundle By Name(cluster=w101, "type"="Lifetime (scan)") -> (w99:T11)
                        n3454 = call "2pparameters.vi"("Params in"=w99, "command"="set") -> ()  [unwired: 1 out]
                      }
                      frame "Lifetime (contour)" {
                        n3455 = local read "Vy-min draw"() -> (w111:dbl)
                        n3456 = local read "Vy-max draw"() -> (w110:dbl)
                        n3457 = local read "Vx-min draw"() -> (w113:dbl)
                        n3458 = local read "Vx-max draw"() -> (w112:dbl)
                        n3459 = local read "xpixels ref"() -> (w109:i32)
                        n3460 = local read "ypixels ref"() -> (w108:i32)
                        n3461 = local read "ROI Type"() -> (w107:u16)
                        n3462 = local read "srateAODOtt"() -> (w118:dbl)
                        n3463 = local read "# of frames"() -> (w123:i32)
                        n3464 = local read "refreshtime"() -> (w115:dbl)
                        n3465 = local read "Pel"() -> (w106:dbl)
                        n3466 = local read "bin"() -> (w121:dbl)
                        n3467 = local read "Override AI buffer"() -> (w104:bool)
                        n3468 = local read "finite samples"() -> (w130:bool)
                        n3469 = local read "srateAODOtt"() -> (w117:dbl)
                        n3470 = local read "srateAODOtt"() -> (w124:dbl)
                        n3471 = local read "continuous"() -> (w129:bool)
                        n3472 = local read "Angle ref"() -> (w114:dbl)
                        n3473 = local read "wavdet"() -> (w131:bool)
                        n3474 = local read "Vx-ref"() -> (w126:dbl)
                        n3475 = local read "Vy-ref"() -> (w128:dbl)
                        n3476 = local read "avpp"() -> (w127:i32)
                        n3477 = call "tt_timeandsamples.vi"("bin"=w121, "refreshtime"=w115, "srateAODOtt"=w118, "tot#ofsamples"=w123) -> ("refreshrate"=w119:dbl, "refreshbuffer"=w120:i32, "timetracecycles"=w125:i32)  [unwired: 5 in]
                        n3478 = local read "bin"() -> (w122:dbl)
                        n3479 = call "2pparameters.vi"("command"="get") -> ("params out"=w134:T11)  [unwired: 1 in]
                        n3480 = Bundle By Name(cluster=w134, "Drawing Mode"=w107, "measpoints"=w123, "tt_cycles"=w125, "refreshbuffer"=w120, "refreshrate"=w119, "Vx-ref"=w126, "Vy-ref"=w128, "srate"=w117, "finite"=w130, "cont"=w129, "wavdet"=w131, "avpp"=w127, "srateAODO"=w124, "bufferAI"=w120, "bin"=w122, "Angle Img"=w114, "Vxminref"=w113, "Vxmaxref"=w112, "Vyminref"=w111, "Vymaxref"=w110, "Xpixels Img"=w109, "Ypixels Img"=w108, "Pel"=w106, "Vz-reset"=0.0, "AIoverride"=w104, "type"="Lifetime (contour)") -> (w132:T11)
                        n3481 = Reciprocal(x=w119) -> (1/x=w116:dbl)
                        n3482 = local write "refreshtime"(w116) -> ()
                        n3483 = call "2pparameters.vi"("Params in"=w132, "command"="set") -> ()  [unwired: 1 out]
                      }
                      frame "X-Y-Z-t movie" {
                      }
                      frame "linescan" {
                      }
                      frame "Timetrace" {
                        n3484 = local read "Vy-min draw"() -> (w144:dbl)
                        n3485 = local read "Vy-max draw"() -> (w143:dbl)
                        n3486 = local read "Vx-min draw"() -> (w146:dbl)
                        n3487 = local read "Vx-max draw"() -> (w145:dbl)
                        n3488 = local read "xpixels ref"() -> (w142:i32)
                        n3489 = local read "ypixels ref"() -> (w141:i32)
                        n3490 = local read "ROI Type"() -> (w140:u16)
                        n3491 = local read "srateAODOtt"() -> (w151:dbl)
                        n3492 = local read "# of frames"() -> (w156:i32)
                        n3493 = local read "refreshtime"() -> (w148:dbl)
                        n3494 = local read "Pel"() -> (w139:dbl)
                        n3495 = local read "bin"() -> (w154:dbl)
                        n3496 = local read "Override AI buffer"() -> (w137:bool)
                        n3497 = local read "finite samples"() -> (w163:bool)
                        n3498 = local read "srateAODOtt"() -> (w150:dbl)
                        n3499 = local read "srateAODOtt"() -> (w157:dbl)
                        n3500 = local read "continuous"() -> (w162:bool)
                        n3501 = local read "Angle ref"() -> (w147:dbl)
                        n3502 = local read "wavdet"() -> (w164:bool)
                        n3503 = local read "Vx-ref"() -> (w159:dbl)
                        n3504 = local read "Vy-ref"() -> (w161:dbl)
                        n3505 = local read "avpp"() -> (w160:i32)
                        n3506 = call "tt_timeandsamples.vi"("bin"=w154, "refreshtime"=w148, "srateAODOtt"=w151, "tot#ofsamples"=w156) -> ("refreshrate"=w152:dbl, "refreshbuffer"=w153:i32, "timetracecycles"=w158:i32)  [unwired: 5 in]
                        n3507 = local read "bin"() -> (w155:dbl)
                        n3508 = call "2pparameters.vi"("command"="get") -> ("params out"=w167:T11)  [unwired: 1 in]
                        n3509 = Bundle By Name(cluster=w167, "Drawing Mode"=w140, "measpoints"=w156, "tt_cycles"=w158, "refreshbuffer"=w153, "refreshrate"=w152, "Vx-ref"=w159, "Vy-ref"=w161, "srate"=w150, "finite"=w163, "cont"=w162, "wavdet"=w164, "avpp"=w160, "srateAODO"=w157, "bufferAI"=w153, "bin"=w155, "Angle Img"=w147, "Vxminref"=w146, "Vxmaxref"=w145, "Vyminref"=w144, "Vymaxref"=w143, "Xpixels Img"=w142, "Ypixels Img"=w141, "Pel"=w139, "Vz-reset"=0.0, "AIoverride"=w137, "type"="Timetrace") -> (w165:T11)
                        n3510 = Reciprocal(x=w152) -> (1/x=w149:dbl)
                        n3511 = local write "refreshtime"(w149) -> ()
                        n3512 = call "2pparameters.vi"("Params in"=w165, "command"="set") -> ()  [unwired: 1 out]
                      }
                      frame "Lifetime (point)" {
                      }
                    }
                  }
                  frame #1 {
                    w170 = FALSE ("wavdet")
                    n3513 = call "2pparameters.vi"("command"="get") -> ("params out"=w174:T11)  [unwired: 1 in]
                    n3514 = Bundle By Name(cluster=w174, "finite"=w170, "cont"=w170, "wavdet"=TRUE) -> (w171:T11)
                    n3515 = call "2pparameters.vi"("Params in"=w171, "command"="set") -> ()  [unwired: 1 out]
                  }
                  frame #2 {
                    # "change active waveform numbers array"
                    n3516 = local read "AO channels"() -> (w181:u32)
                    n3517 = call "2pparameters.vi"("command"="get") -> ("params out"=w179:T11)  [unwired: 1 in]
                    n3518 = in-place {
                      in-place-border: w181 -> [w185]
                      in-place-border: [w182] -> w176
                      n3519 = in-place-cluster #49(w179) -> ("aAO"=w184:u32[])
                      n3520 = call "add channel to active arrayv2.vi"("line array in"=w184, "line to add"=w185) -> ("line array out"=w183:u32[], "addition"=w182:bool)  [unwired: 1 out]
                      n3521 = in-place-cluster #49("aAO"=w183) -> (w177:T11)
                    }
                    n3522 = local write "addAO"(w176) -> ()
                    n3523 = call "2pparameters.vi"("Params in"=w177, "command"="set") -> ()  [unwired: 1 out]
                  }
                  frame #3 {
                    # "update GUI"
                    n3524 = local read "addAO"() -> (w186:bool)
                    n3525 = case shown="True" w186 {
                      frame False {
                      }
                      frame True {
                        n3526 = call "Used AO lines.vi"() -> ("used AO names"=w190:string[], "used AO lines"=w192:tag[])  [unwired: 2 in]
                        n3527 = control-ref of="Analog Lines Plot"() -> (w191:refnum<vi>)
                        n3528 = control-ref of="Digital Lines Plot"() -> (w189:refnum<vi>)
                        n3529 = call "Used DO lines.vi"() -> ("used DO names"=w188:string[], "used DO lines"=w187:tag[])  [unwired: 2 in]
                        n3530 = local write "Analog Used Lines"(w192) -> ()
                        n3531 = local write "Analog Used Names"(w190) -> ()
                        n3532 = local write "Digital Used Lines"(w187) -> ()
                        n3533 = local write "Digital Used Names"(w188) -> ()
                        n3534 = call "prepDOWaveplot.vi"("DigitalGraph in"=w189, "used DO names"=w188) -> ()  [unwired: 1 in]
                        n3535 = call "prepAOWaveplot.vi"("WaveformGraph in"=w191, "Analog Used Names"=w190) -> ()  [unwired: 1 in]
                      }
                    }
                  }
                  frame #4 {
                    n3536 = local read "addAO"() -> (w193:bool)
                    n3537 = case shown="True" w193 {
                      frame False {
                      }
                      frame True {
                        # "add parameters\nto parameter array"
                        n3538 = local read "Build analog waveform tabs"() -> (w194:enum32{"Square", "Triangle", "Matlab"})
                        n3539 = case shown="\"Square\", Default" w194 {
                          frame "Square", Default {
                            w207 = 0.0 ("Offset (V)")
                            n3540 = local read "Meastab"() -> (w196:enum32{"X-Y Image", "Linescan", "Timetrace"})
                            n3541 = call "waveformparamsv2.vi"("command"="get") -> ("Params out"=w205:T15)  [unwired: 4 in, 2 out]
                            n3542 = Unbundle By Name(w205) -> ("AO parameters"=w202:T16)
                            n3543 = case shown="\"Timetrace\"" w196 {
                              tunnel: [w218 w219] -> w195
                              frame "X-Y Image", Default {
                                n3544 = local read "Sampling rate"() -> (w218:dbl)
                              }
                              frame "Timetrace" {
                                n3545 = local read "srateAODOtt"() -> (w219:dbl)
                              }
                            }
                            n3546 = local read "Start amplitude (V)"() -> (w215:dbl)
                            n3547 = local read "phase shift (ms)"() -> (w208:dbl)
                            n3548 = local read "Step size (V)"() -> (w213:dbl)
                            n3549 = local read "Baseline (V)"() -> (w214:dbl)
                            n3550 = local read "Period (ms)"() -> (w211:dbl)
                            n3551 = local read "padding value"() -> (w198:dbl)
                            n3552 = local read "Repeats"() -> (w217:dbl)
                            n3553 = local read "DC (%)"() -> (w212:dbl)
                            n3554 = local read "Cycles"() -> (w216:dbl)
                            n3555 = local read "Pulses"() -> (w209:dbl)
                            n3556 = Index Array(array=w202, index=0) -> (element=w203:T17)
                            n3557 = Bundle By Name(cluster=w203, "AOtab"=0.0 ("Repeats"), "Repeats"=w217, "Cycles"=w216, "Start amplitude (V)"=w215, "Baseline (V)"=w214, "Step size (V)"=w213, "DC (%)"=w212, "Sampling frequency (Hz)"=w195, "Period (ms)"=w211, "Offset (V)"=w207, "Amplitude (V)"=w207, "Frequency"=w207, "Tri Repeats"=w207, "phase shift (ms)"=w208, "Pulses"=w209, "Matlab wave file"=path "", "padding value"=w198) -> (w200:T17)
                            n3558 = Build Array(w200) -> (w199:T16)
                            n3559 = call "waveformparamsv2.vi"("command"="add AO", "add AO"=w199) -> ()  [unwired: 3 in, 3 out]
                          }
                          frame "Matlab" {
                            w225 = 0.0 ("Repeats")
                            n3560 = local read "Meastab"() -> (w221:enum32{"X-Y Image", "Linescan", "Timetrace"})
                            n3561 = call "waveformparamsv2.vi"("command"="get") -> ("Params out"=w232:T15)  [unwired: 4 in, 2 out]
                            n3562 = Unbundle By Name(w232) -> ("AO parameters"=w229:T16)
                            n3563 = case shown="\"Timetrace\"" w221 {
                              tunnel: [w235 w236] -> w220
                              frame "X-Y Image", Default {
                                n3564 = local read "Sampling rate"() -> (w235:dbl)
                              }
                              frame "Timetrace" {
                                n3565 = local read "srateAODOtt"() -> (w236:dbl)
                              }
                            }
                            n3566 = local read "Matlab waveform path"() -> (w222:path)
                            n3567 = local read "Matlab padding value"() -> (w224:dbl)
                            n3568 = Index Array(array=w229, index=0) -> (element=w230:T17)
                            n3569 = call "matlabwfexistsdialogue.vi"("Matlab waveform path"=w222) -> ("mtalab waveform path out"=w223:path)
                            n3570 = Bundle By Name(cluster=w230, "AOtab"=2.0 ("Repeats"), "Repeats"=w225, "Cycles"=w225, "Start amplitude (V)"=w225, "Baseline (V)"=w225, "Step size (V)"=w225, "DC (%)"=w225, "Sampling frequency (Hz)"=w220, "Period (ms)"=w225, "Offset (V)"=w225, "Amplitude (V)"=w225, "Frequency"=w225, "Tri Repeats"=w225, "phase shift (ms)"=w225, "Pulses"=w225, "Matlab wave file"=w223, "padding value"=w224) -> (w227:T17)
                            n3571 = Build Array(w227) -> (w226:T16)
                            n3572 = call "waveformparamsv2.vi"("command"="add AO", "add AO"=w226) -> ()  [unwired: 3 in, 3 out]
                          }
                          frame "Triangle" {
                            w242 = 0.0 ("Offset (V)")
                            n3573 = local read "Meastab"() -> (w238:enum32{"X-Y Image", "Linescan", "Timetrace"})
                            n3574 = call "waveformparamsv2.vi"("command"="get") -> ("Params out"=w254:T15)  [unwired: 4 in, 2 out]
                            n3575 = Unbundle By Name(w254) -> ("AO parameters"=w251:T16)
                            n3576 = case shown="\"Timetrace\"" w238 {
                              tunnel: [w256 w257] -> w237
                              frame "X-Y Image", Default {
                                n3577 = local read "Sampling rate"() -> (w256:dbl)
                              }
                              frame "Timetrace" {
                                n3578 = local read "srateAODOtt"() -> (w257:dbl)
                              }
                            }
                            n3579 = local read "Tri padding value"() -> (w240:dbl)
                            n3580 = local read "Amplitude (V)"() -> (w245:dbl)
                            n3581 = local read "Tri Phase (s)"() -> (w241:dbl)
                            n3582 = local read "Tri Repeats"() -> (w243:dbl)
                            n3583 = local read "Frequency"() -> (w244:dbl)
                            n3584 = local read "Offset (V)"() -> (w246:dbl)
                            n3585 = Index Array(array=w251, index=0) -> (element=w252:T17)
                            n3586 = Bundle By Name(cluster=w252, "AOtab"=1.0 ("Repeats"), "Repeats"=w242, "Cycles"=w242, "Start amplitude (V)"=w242, "Baseline (V)"=w242, "Step size (V)"=w242, "DC (%)"=w242, "Sampling frequency (Hz)"=w237, "Period (ms)"=w242, "Offset (V)"=w246, "Amplitude (V)"=w245, "Frequency"=w244, "Tri Repeats"=w243, "phase shift (ms)"=w242, "Pulses"=w242, "Matlab wave file"=path "", "Tri phase"=w241, "padding value"=w240) -> (w249:T17)
                            n3587 = Build Array(w249) -> (w248:T16)
                            n3588 = call "waveformparamsv2.vi"("command"="add AO", "add AO"=w248) -> ()  [unwired: 3 in, 3 out]
                          }
                        }
                      }
                    }
                  }
                  frame #5 {
                    n3589 = local read "addAO"() -> (w258:bool)
                    n3590 = case shown="True" w258 {
                      frame False {
                      }
                      frame True {
                        # "add waveform to waveform array; correct waveform lengths and plot"
                        n3591 = local read "Meastab"() -> (w262:enum32{"X-Y Image", "Linescan", "Timetrace"})
                        n3592 = local read "Build analog waveform tabs"() -> (w272:enum32{"Square", "Triangle", "Matlab"})
                        n3593 = case shown="\"Timetrace\"" w262 {
                          tunnel: [w280 w281] -> w261
                          frame "X-Y Image", Default {
                            n3594 = local read "Sampling rate"() -> (w280:dbl)
                          }
                          frame "Timetrace" {
                            n3595 = local read "srateAODOtt"() -> (w281:dbl)
                          }
                        }
                        n3596 = call "waveformparamsv2.vi"("command"="get last AO") -> ("last AO"=w274:T17)  [unwired: 4 in, 2 out]
                        n3597 = case shown="\"Matlab\"" w272 {
                          tunnel: w274 -> [w284 w286 w288]
                          tunnel: [w283 w285 w287] -> w273
                          frame "Square", Default {
                            n3598 = call "generateRampedSquareWave_fromAOparameters.vi"("AO params"=w284) -> ("Waveform"=w283:waveform(dbl))  [unwired: 1 out]
                          }
                          frame "Triangle" {
                            n3599 = call "generateTriWave_fromAOparameters.vi"("AO params"=w286) -> ("Waveform"=w285:waveform(dbl))  [unwired: 1 out]
                          }
                          frame "Matlab" {
                            n3600 = call "matlabAOwffromparam.vi"("Cluster"=w288) -> ("Waveform"=w287:waveform(dbl))  [unwired: 1 out]
                          }
                        }
                        n3601 = property on="refwf" class="Ring (strict)"() -> ("RingText.Text"=w265:string)  [unwired: 2 in, 2 out]
                        n3602 = call "waveformsAObuffer.vi"("command"="get") -> ("AO wf out"=w278:waveform(dbl)[])  [unwired: 1 in]
                        n3603 = Build Array (concatenate)(w278, w273) -> (w275:waveform(dbl)[])
